vi "Schedule Logger.vi"   [LabVIEW 2020, in "Schedule Modul.lvlib"]
uses:
  Schedule Modul.lvlib
  Allgemein/allgemeine Sub-VIs.lvlib
  Aktion FGV Schedule Log.ctl
panel:
  # "Schedule in Datei loggen!"
types:
  T1 = typedef "Schedule Modul.lvlib/Aktion FGV Schedule Log.ctl" = enum16{"lesen", "neuer Eintrag", "laden", "löschen", "Anzeige löschen"}
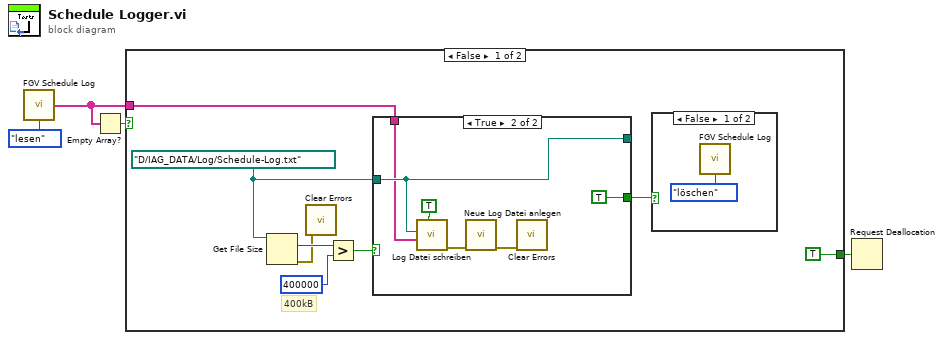
[diagram p0: block diagram]
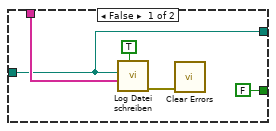
[diagram p3: hidden frame]
diagram:
  n1 = call "FGV Schedule Log.vi"("Aktion"=Aktion_FGV_Schedule_Log."lesen") -> ("Log Array"=w1:string[])  [unwired: 11 in, 3 out]
  n2 = Empty Array?(array=w1) -> (empty?=w3:bool)
  n3 = case shown="False" w3 {
    tunnel: w1 -> [w7 _]
    tunnel: [TRUE _] -> w4
    frame False {
      w9 = path "D:/IAG_DATA/Log/Schedule-Log.txt" ("Datei")
      # "400kB"
      n4 = Get File Size(file=w9) -> (size (in bytes)=w10:i64, 0:w8:errorcluster)  [unwired: 1 in, 1 out]
      n5 = call <vilib>:"Clear Errors.vi"("error in (no error)"=w8) -> ()  [unwired: 5 in, 2 out]
      n6 = Greater?(x=w10, y=i64 400000) -> (0:w12:bool)
      n7 = case shown="True" w12 {
        tunnel: w7 -> [w18 w20]
        tunnel: w9 -> [w16 w23]
        tunnel: [w16 w23] -> _
        tunnel: [FALSE TRUE] -> w5
        frame False {
          n8 = call "Log Datei schreiben.vi"("An Datei Anhängen?"=TRUE, "Array"=w18, "Dateipfad"=w16) -> ("error out"=w14:errorcluster)  [unwired: 8 in]
          n9 = call <vilib>:"Clear Errors.vi"("error in (no error)"=w14) -> ()  [unwired: 5 in, 2 out]
        }
        frame True {
          n10 = call "Log Datei schreiben.vi"("An Datei Anhängen?"=TRUE, "Array"=w20, "Dateipfad"=w23) -> ("error out"=w22:errorcluster)  [unwired: 8 in]
          n11 = call "Neue Log Datei anlegen.vi"("error in (no error)"=w22) -> ("error out"=w19:errorcluster)  [unwired: 10 in]
          n12 = call <vilib>:"Clear Errors.vi"("error in (no error)"=w19) -> ()  [unwired: 5 in, 2 out]
        }
      }
      n13 = case shown="False" w5 {
        frame False {
          n14 = call "FGV Schedule Log.vi"("Aktion"=Aktion_FGV_Schedule_Log."löschen") -> ()  [unwired: 11 in, 4 out]
        }
        frame True {
        }
      }
    }
    frame True {
    }
  }
  n15 = Request Deallocation(w4) -> ()
